vi "Translate_ARRAY.vi"(8 "error IN":errorcluster, 10 "Cle":string, 11 "Arr Refnum":refnum<vi>) -> (0 "error out":errorcluster)   [LabVIEW 2011]
uses:
  Dictionnary/EnumCommandDictionnaire.ctl
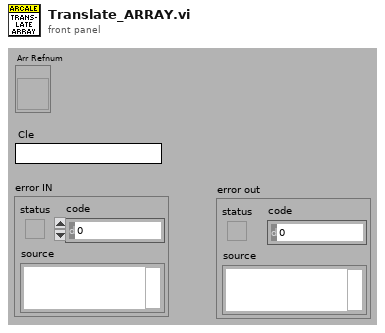
[diagram p1: front panel]
types:
  T1 = typedef "EnumCommandDictionnaire.ctl" = enum16{"Load", "Translate", "Save", "GetDico", "Set : A traduire = Vrai", "Set : A Traduire = Faux", "SetDico"}
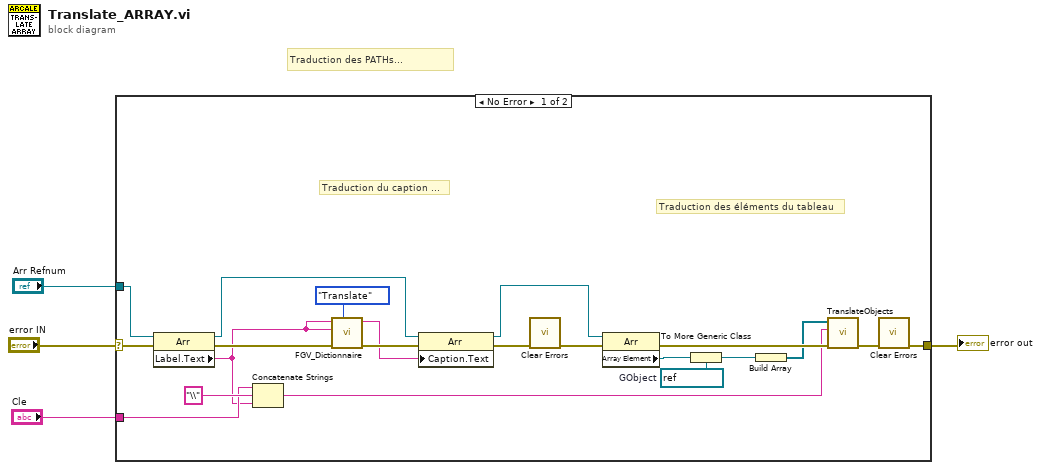
[diagram p0: block diagram]
diagram:
  # "Traduction des PATHs..."
  n1 = case shown="No Error" "error IN" {
    selector: "error IN" -> [w25 w26]
    tunnel: "Arr Refnum" -> [w24 _]
    tunnel: "Cle" -> [w22 _]
    tunnel: [w6 w26] -> w1
    frame No Error {
      w13 = refnum<vi> refnum  # GObject
      # "Traduction des éléments du tableau"
      # "Traduction du caption ..."
      n2 = property class="Arr"(reference=w24, error in=w25) -> (reference out=w21:refnum<vi>, error out=w11:errorcluster, "Label.Text"=w5:string)
      n3 = Concatenate Strings(w22, "\\" ("string"), w5) -> (w9:string)
      n4 = call "FGV_Dictionnaire.vi"("Command"=EnumCommandDictionnaire."Translate", "error in (no error)"=w11, "Chaîne"=w5, "Clé"=w5) -> ("error out"=w10:errorcluster, "Traduction"=w8:string)  [unwired: 5 in, 1 out]
      n5 = property class="Arr"(reference=w21, error in=w10, "Caption.Text"=w8) -> (reference out=w19:refnum<vi>, error out=w20:errorcluster)
      n6 = call <vilib>:"Clear Errors.vi"("error in (no error)"=w20) -> ("error out"=w7:errorcluster)  [unwired: 6 in]
      n7 = property class="Arr"(reference=w19, error in=w7) -> (error out=w17:errorcluster, "Array Element"=w18:refnum<vi>)  [unwired: 1 out]
      n8 = To More Generic Class(target class=w13, reference=w18) -> (generic class reference=w14:refnum<vi>)
      n9 = Build Array(w14) -> (w15:refnum<vi>[])
      n10 = call "TranslateObjects.vi"("errorIN"=w17, "Cle"=w9, "AllObjs[]In"=w15) -> ("error out"=w16:errorcluster)  [unwired: 7 in, 1 out]
      n11 = call <vilib>:"Clear Errors.vi"("error in (no error)"=w16) -> ("error out"=w6:errorcluster)  [unwired: 6 in]
    }
    frame Error {
    }
  }
  "error out" <- w1
